vi "Read Binary Config.vi"(4 "Class Name is Included":bool, 6 "byte order (0:big-endian, network order)":T1(ring), 8 "error in (no error)":errorcluster, 10 "Binary":string, 11 "Subset_STR in":refnum<class "Subset_STR.lvclass">) -> (0 "error out":errorcluster, 2 "Remaining":string, 3 "Subset_STR out":refnum<class "Subset_STR.lvclass">)   [LabVIEW 2021, in "Subset_STR.lvclass"]
uses:
  Subset_STR.lvclass
  Subset_STR.lvclass/Subset_STR.ctl
  Abs_Types/String/Abs_String.lvclass
  Abs_Types/Numeric/Abs_Numeric.lvclass
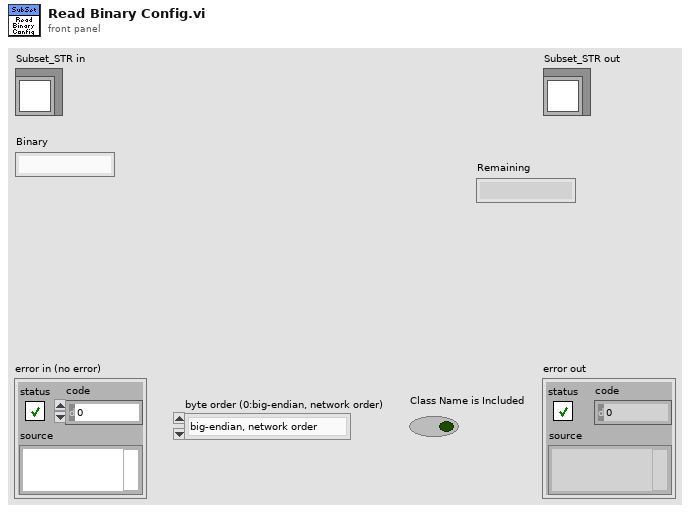
[diagram p1: front panel]
types:
  T1 = enum16{"big-endian, network order", "native, host order", "little-endian"}
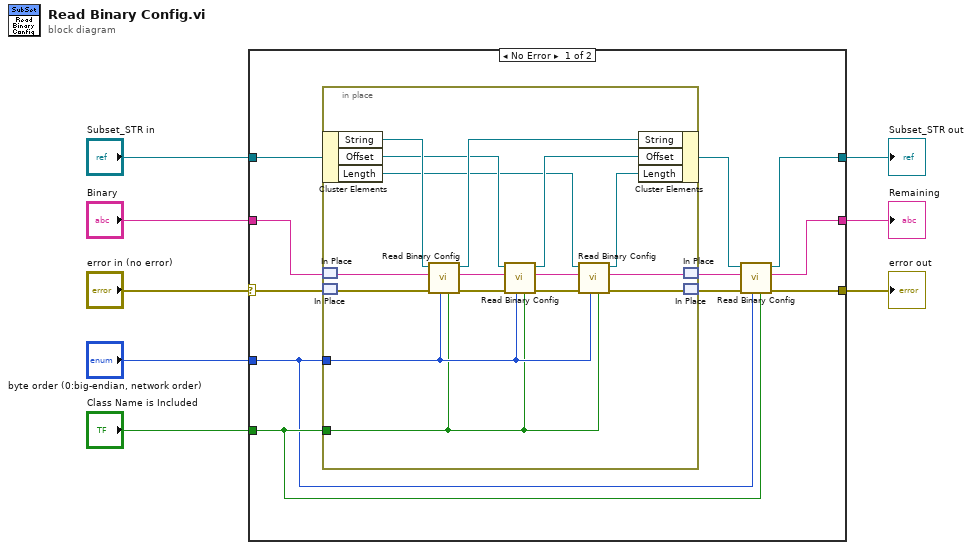
[diagram p0: block diagram]
diagram:
  n1 = case shown="No Error" "error in (no error)" {
    selector: "error in (no error)" -> [w18 w36]
    tunnel: "Subset_STR in" -> [w19 w38]
    tunnel: [w16 w36] -> w6
    tunnel: [w14 w38] -> w5
    tunnel: "Binary" -> [w12 w37]
    tunnel: [w11 w37] -> w3
    tunnel: "Class Name is Included" -> [w10 _]
    tunnel: "byte order (0:big-endian, network order)" -> [w9 _]
    frame No Error {
      n2 = in-place {
        in-place-border: w9 -> [w21]
        in-place-border: w10 -> [w20]
        n3 = in-place-cluster #1(w19) -> ("String"=w34:refnum<class "Abs_String.lvclass">, "Offset"=w29:refnum<class "Abs_Numeric.lvclass">, "Length"=w25:refnum<class "Abs_Numeric.lvclass">)
        n4 = in-place-match #2(w12) -> (w33:string)
        n5 = in-place-match #3(w18) -> (w35:errorcluster)
        n6 = call-dynamic "Read Binary Config.vi"("Class Name is Included"=w20, "byte order (0:big-endian, network order)"=w21, "error in (no error)"=w35, "Binary"=w33, "Abs_Type in"=w34) -> ("error out"=w31:errorcluster, "Remaining"=w32:string, "Abs_Type out"=w30:refnum<class "Abs_String.lvclass">)  [unwired: 4 in]
        n7 = call-dynamic "Read Binary Config.vi"("Class Name is Included"=w20, "byte order (0:big-endian, network order)"=w21, "error in (no error)"=w31, "Binary"=w32, "Abs_Type in"=w29) -> ("error out"=w27:errorcluster, "Remaining"=w26:string, "Abs_Type out"=w28:refnum<class "Abs_Numeric.lvclass">)  [unwired: 4 in]
        n8 = call-dynamic "Read Binary Config.vi"("Class Name is Included"=w20, "byte order (0:big-endian, network order)"=w21, "error in (no error)"=w27, "Binary"=w26, "Abs_Type in"=w25) -> ("error out"=w22:errorcluster, "Remaining"=w23:string, "Abs_Type out"=w24:refnum<class "Abs_Numeric.lvclass">)  [unwired: 4 in]
        n9 = in-place-cluster #1("String"=w30, "Offset"=w28, "Length"=w24) -> (w15:refnum<class "Subset_STR.lvclass">)
        n10 = in-place-match #2(w23) -> (w13:string)
        n11 = in-place-match #3(w22) -> (w17:errorcluster)
      }
      n12 = call-parent "Read Binary Config.vi"("Class Name is Included"=w10, "byte order (0:big-endian, network order)"=w9, "error in (no error)"=w17, "Binary"=w13, "Abs_Type in"=w15) -> ("error out"=w16:errorcluster, "Remaining"=w11:string, "Abs_Type out"=w14:refnum<class "Subset_STR.lvclass">)  [unwired: 4 in]
    }
    frame Error {
    }
  }
  "error out" <- w6
  "Subset_STR out" <- w5
  "Remaining" <- w3
